vi "全局.vi"() -> ()   [LabVIEW 2016]
panel:
  out "Image":T1(plugin-control)
  out "Exit":bool
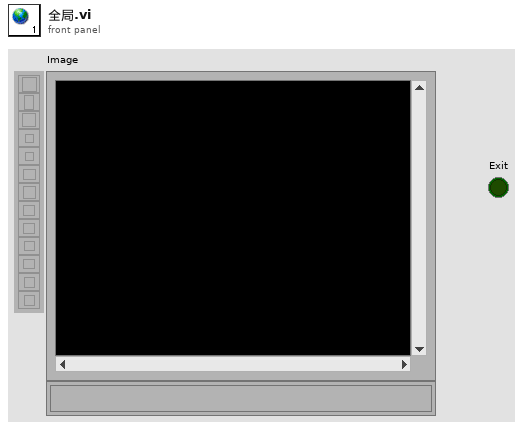
[diagram p1: front panel]
types:
  T1 = typedef "IMAQ Image.ctl" = refnum<image>
diagram:
